vi "RVC 3-link serial robot Primatic Modified DH.vi"() -> ()   [LabVIEW 2014]
uses:
  <vilib>/Analysis/Matrix/Datatypes/RealMatrix.ctl
  <vilib>/robotics/Kinematics/Analytical/Initialize Generic Serial Arm.vi
  <vilib>/robotics/Kinematics/Analytical/NI_Robotics_AnalyticKinematics.lvlib
  <vilib>/robotics/Kinematics/Robot/NI_Robotics_Serial Robot Arm.lvclass
  <vilib>/Analysis/Matrix/NI_Matrix.lvlib
panel:
  in  "appended array":dbl[](array[numeric])=[0.2, 0.30000000000000004, 0.30000000000000004]
  out "transformation":picture
  out "forward kinematics":T1
  out "3D Picture":refnum<vi>(3d-picture)
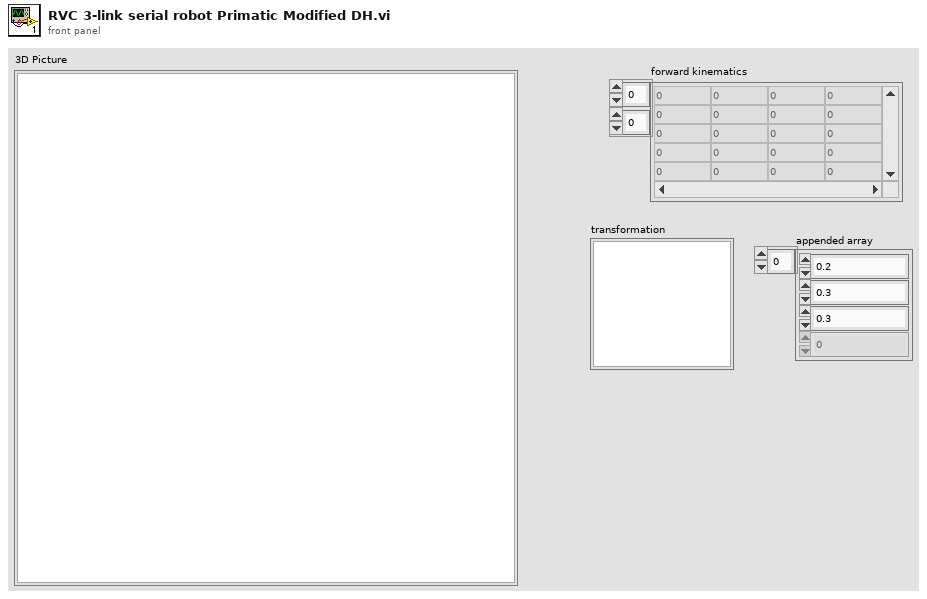
[diagram p1: front panel]
types:
  T1 = typedef "NI_Matrix.lvlib/RealMatrix.ctl" = dbl[][]
  T2 = typedef "DH Kinematic Parameters.ctl" = cluster{"twist angle":dbl, "length":dbl, "rotation angle":dbl, "offset distance":dbl, "joint type":T3, "joint coordinate offset":dbl}
  T3 = typedef "NI_Robotics_Link.lvclass/Joint Type.ctl" = enum16{"Revolute", "Prismatic"}
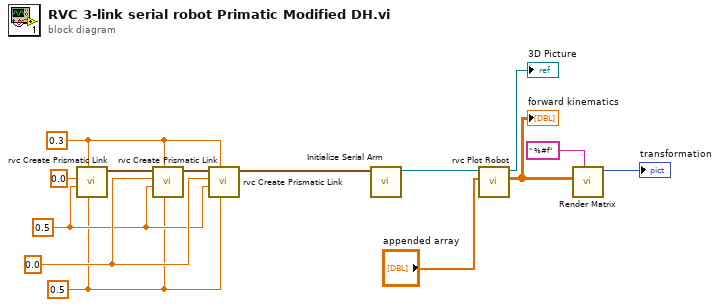
[diagram p0: block diagram]
diagram:
  w2 = 0.5 ("offset distance (d)")
  w4 = 0.3 ("rotation angle (theta)")
  w3 = 0.5 ("rotation angle (theta)")
  w5 = 0.0 ("length (a)")
  n1 = call "rvc Create Prismatic Link.vi"("offset distance (d)"=w2, "rotation angle (theta)"=w4, "twist angle (alpha)"=w3, "length (a)"=0.0) -> ("Array"=w6:T2[])  [unwired: 7 in]
  n2 = call "rvc Create Prismatic Link.vi"("offset distance (d)"=w2, "rotation angle (theta)"=w4, "twist angle (alpha)"=w3, "length (a)"=w5, "Array 2"=w6) -> ("Array"=w8:T2[])  [unwired: 6 in]
  n3 = call "rvc Create Prismatic Link.vi"("offset distance (d)"=w2, "rotation angle (theta)"=w4, "twist angle (alpha)"=w3, "length (a)"=w5, "Array 2"=w8) -> ("Array"=w7:T2[])  [unwired: 6 in]
  n4 = call-poly <vilib>:"Initialize Serial Arm.vi"("kinematic parameters"=w7) -> ("serial arm out"=w14:refnum<class "NI_Robotics_Serial Robot Arm.lvclass">)  [unwired: 9 in, 1 out]
  n5 = call "rvc Plot Robot.vi"("joint positions"="appended array", "NI_Robotics_Serial Robot Arm in"=w14) -> ("forward kinematics"=w10:T1, "Scene Object Out"=→"3D Picture":refnum<vi>)  [unwired: 7 in, 1 out]
  "forward kinematics" <- w10
  n6 = call "Render Matrix.vi"("format string"=" %#f", "A"=w10) -> ("picture out"=→"transformation":picture)  [unwired: 9 in]
